vi "Robot Global Data.vi"() -> ()   [LabVIEW 2016]
doc: "This global VI can contain as many global variables as you need. Place a control on the panel, give it a good name. To read or write to it from a VI, drag the icon to the diagram of that VI. You can also drag from the project. Click on the node to change which global you access. You shouldn't have multiple locations writing to a global or it will cause a race-condition."
uses:
  <vilib>/Rock Robotics/WPI/Camera/WPI_CameraImageSize.ctl
  <vilib>/Rock Robotics/WPI/DriverStation/WPI_DriverStationRobotMode2.ctl
panel:
  out "Shift?":bool
  out "PID?":bool
  out "TimeElapsed":dbl
  out "pprate1":dbl
  out "pprate0":dbl
  out "PathPlanningv1":dbl[][](array[numeric])
  out "Pitch":dbl
  out "Roll":dbl
  out "Yaw":dbl
  out "LinearAcceleration Z":dbl
  out "LinearAcceleration Y":dbl
  out "LinearAcceleration X":dbl
  out "Displacement Z":dbl
  out "Displacement Y":dbl
  out "Displacement X":dbl
  out "Velocity Z":dbl
  out "Velocity Y":dbl
  out "Velocity X":dbl
  in  "TargetsFound":bool
  out "Mid":dbl
  in  "AvgMid":dbl[](array[numeric])
  out "temp":dbl=-1.0
  out "GearAdjustValue":dbl=50.0
  out "GearAdjust":bool
  out "Rate1":dbl
  out "Rate0":dbl
  in  "Robot Mode":T1
  in  "image size":T2=enum."320x240"
  in  "Enable Vision":bool
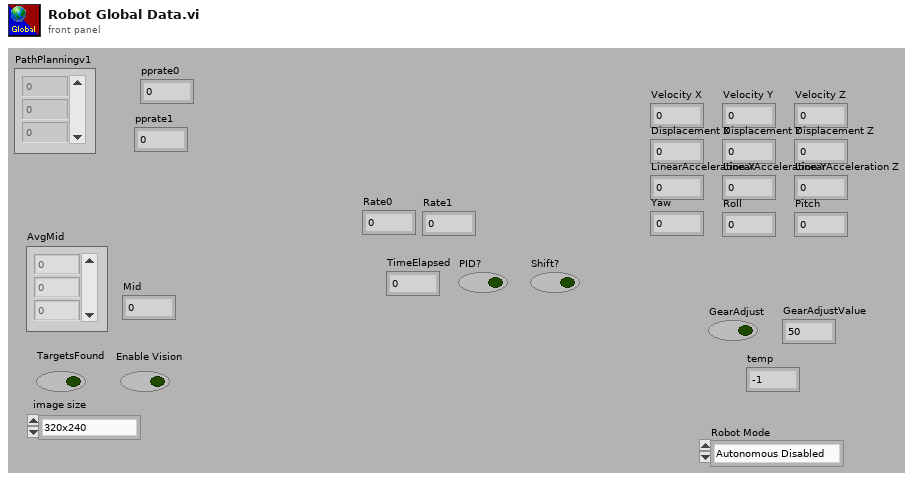
[diagram p1: front panel]
types:
  T1 = typedef "WPI_DriverStationRobotMode2.ctl" = enum16{"Autonomous Disabled", "Autonomous Enabled", "Teleop Disabled", "Teleop Enabled", "Disconnected", "Finish", "Test Disabled", "Test Enabled", "Emergency Stopped"}
  T2 = typedef "WPI_CameraImageSize.ctl" = enum16{"640x480", "320x240", "160x120", "Custom"}
diagram:
